vi "Write Section.vi"(8 "Error In":errorcluster, 9 "Section":string, 10 "Data":string, 11 "Path":path) -> (0 "Error Out":errorcluster)   [LabVIEW 2017, in "Configit.lvlib"]
uses:
  Configit.lvlib
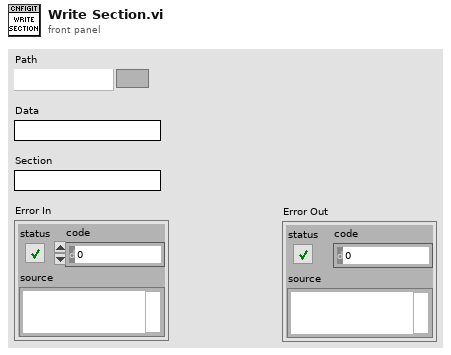
[diagram p1: front panel]
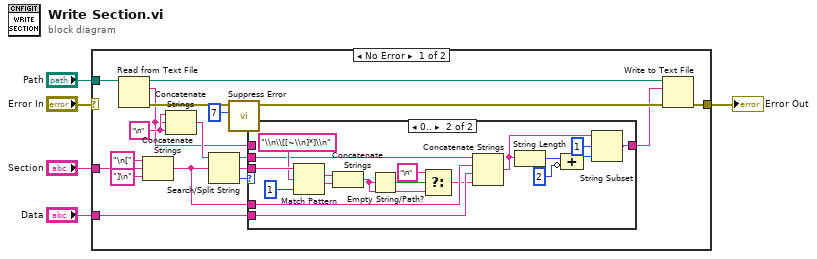
[diagram p0: block diagram]
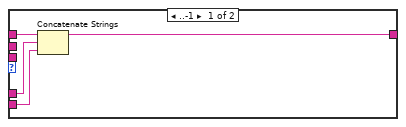
[diagram p2: hidden frame]
diagram:
  n1 = case shown="No Error" "Error In" {
    selector: "Error In" -> [_ w45]
    tunnel: "Path" -> [w6 _]
    tunnel: [w12 w45] -> w4
    tunnel: "Section" -> [w14 _]
    tunnel: "Data" -> [w10 _]
    frame No Error {
      w13 = "\n" ("string")
      n2 = Read from Text File(file (use dialog)=w6) -> (text=w7:string, error out=w17:errorcluster)  [unwired: 1 in, 4 out]
      n3 = Concatenate Strings("\n[" ("string"), w14, "]\n" ("string")) -> (w18:string)
      n4 = Concatenate Strings(w13, w7, w13) -> (w20:string)
      n5 = Search/Split String(string=w20, search string/char (-)=w18) -> (substring before match=w9:string, match + rest of string=w19:string, offset of match=w11:i32)  [unwired: 1 in]
      n6 = call "Suppress Error.vi"("Error Code"=7, "Error In"=w17) -> ("Error Out"=w15:errorcluster)  [unwired: 4 in, 1 out]
      n7 = case shown="0.." w11 {
        tunnel: w19 -> [_ w43]
        tunnel: w18 -> [w25 w35]
        tunnel: w10 -> [w24 w34]
        tunnel: w9 -> [_ w36]
        tunnel: [w23 w27] -> w8
        tunnel: w7 -> [w26 _]
        frame ..-1 {
          n8 = Concatenate Strings(w26, w25, w24) -> (w23:string)
        }
        frame 0.. {
          n9 = Match Pattern(string=w43, regular expression="\\n\\[[~\\n]*]\\n", offset (0)=1) -> (match substring=w39:string, after substring=w38:string)  [unwired: 2 out]
          n10 = Concatenate Strings(w39, w38) -> (w41:string)
          n11 = Empty String/Path?(string/path=w41) -> (empty?=w40:bool)
          n12 = Select(t="\n" ("string"), s=w40, f=w41) -> (s? t:f=w33:string)
          n13 = Concatenate Strings(w36, w35, w34, w33) -> (w31:string)
          n14 = String Length(string=w31) -> (length=w30:i32)
          n15 = Compound Arithmetic op=ADD(w30, invert 2 ("value")) -> (w29:i32)
          n16 = String Subset(string=w31, offset (0)=1, length (rest)=w29) -> (substring=w27:string)
        }
      }
      n17 = Write to Text File(file (use dialog)=w6, text=w8, error in=w15) -> (error out=w12:errorcluster)  [unwired: 1 in, 2 out]
    }
    frame Error {
    }
  }
  "Error Out" <- w4
